vi "Configure Current Slew.vi"(8 "error in":errorcluster, 9 "Slew":dbl=0.001 min=0.001 max=9.999 step=0.001, 10 "Slew Type":u16(ring) caption="Type" items=["Negative", "Positive"], 11 "VISA resource name":refnum<visa-resource-name>) -> (0 "error out":errorcluster, 3 "VISA resource name out":refnum<visa-resource-name>)   [LabVIEW 2018, in "IT-M3100.lvlib"]
doc: "This command sets the under-current warm-up time of the power supply.\n<b>Type</b>\n0:Negative\n1:Positive\n<b>Slew</b>\n0.001-9.999"
uses:
  IT-M3100.lvlib
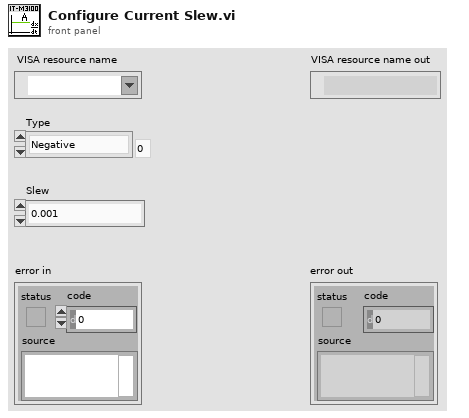
[diagram p1: front panel]
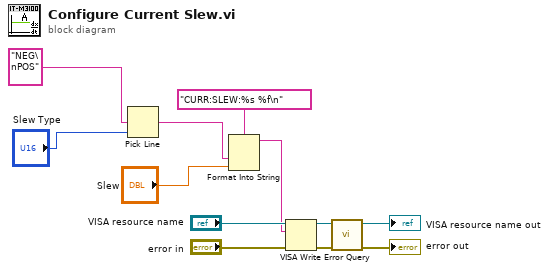
[diagram p0: block diagram]
diagram:
  n1 = Pick Line(multi-line string="NEG\nPOS", line index="Slew Type") -> (output string=w1:string)  [unwired: 1 in]
  n2 = Format Into String(format string="CURR:SLEW:%s %f\n", w1, "Slew") -> (resulting string=w5:string)  [unwired: 2 in, 1 out]
  n3 = VISA Write(VISA resource name="VISA resource name", write buffer=w5, error in (no error)="error in") -> (VISA resource name out=w9:refnum<visa-resource-name>, error out=w10:errorcluster)  [unwired: 1 out]
  n4 = call "Error Query.vi"("error in"=w10, "VISA resource name"=w9) -> ("error out"=→"error out":errorcluster, "VISA resource name out"=→"VISA resource name out":refnum<visa-resource-name>)  [unwired: 6 in, 2 out]
